vi "tester CE14(APIs).vi"() -> ()   [LabVIEW 2018, in "CE14_eMIC.lvlib"]
uses:
  CE14_eMIC.lvlib
  <vilib>/ErrorRing/Error Ring.xnode
panel:
  out "log":string
  out "output 1":dbl
  out "kvar (x.xxxx*kvar)":string
  out "kW (x.xxxx*kW)":string
  out "PF(x.xxx)":string
  out "freq (xx.xxHz)":string
  out "voltage(xxx.xx*V)":string
  out "Current (x.xx Amps)":string
  in  "VISA resource name":refnum<visa-resource-name>="COM12"
  out "success":bool
  in  "kvar":bool
  in  "kW":bool
  in  "pf":bool
  in  "Freq":bool
  in  "voltage":bool
  in  "curr":bool
  in  "stop":bool
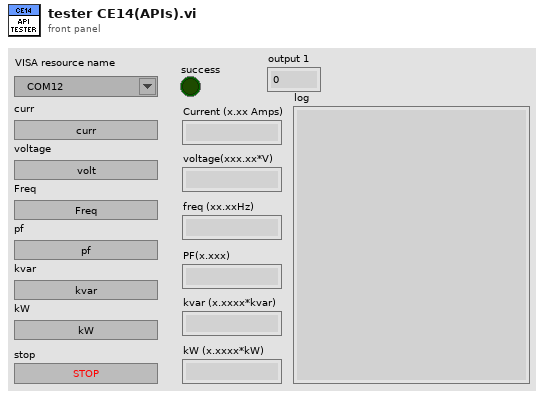
[diagram p1: front panel]
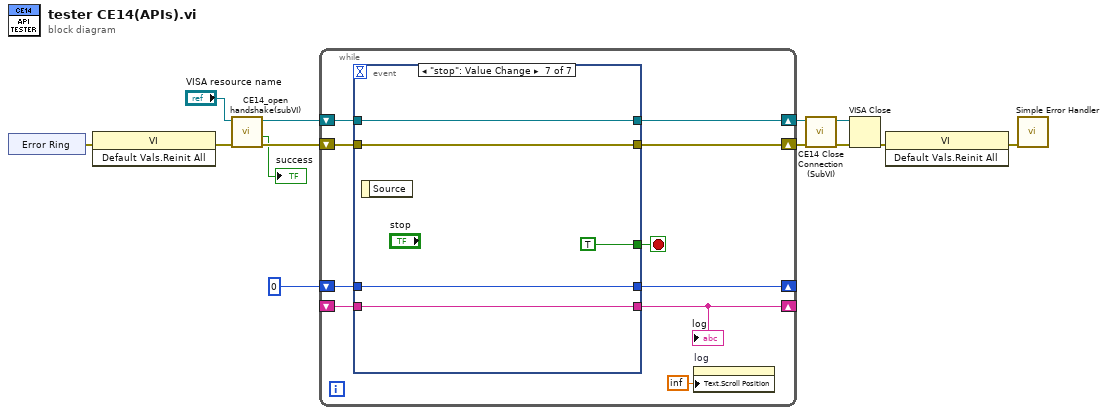
[diagram p0: block diagram]
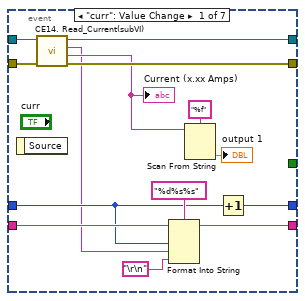
[diagram p2: hidden frame]
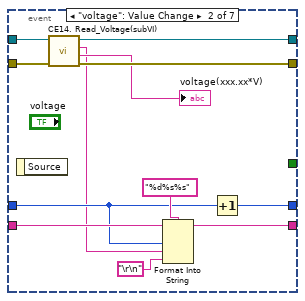
[diagram p3: hidden frame]
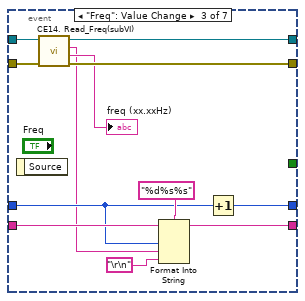
[diagram p4: hidden frame]
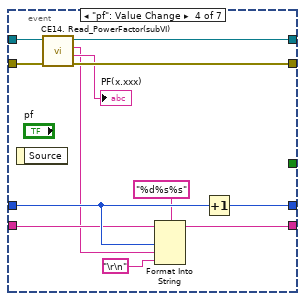
[diagram p5: hidden frame]
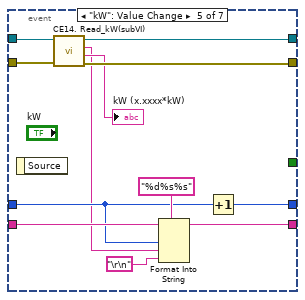
[diagram p6: hidden frame]
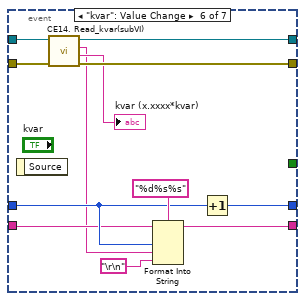
[diagram p7: hidden frame]
diagram:
  n1 = xnode "Error Ring"() -> ("error out"=w13:errorcluster)
  n2 = invoke class="VI" method="Default Vals.Reinit All"(error in=w13) -> (error out=w11:errorcluster)  [unwired: 2 in, 2 out]
  n3 = call "CE14_open handshake(subVI).vi"("error in(no error)"=w11, "VISA resource name"="VISA resource name") -> ("error out"=w10:errorcluster, "success"=→"success":bool, "VISA resource name 2"=w9:refnum<visa-resource-name>)  [unwired: 6 in, 1 out]
  n4 = while {
    shift-right: [w22] -> w6
    shift-left: w10 -> [w23]
    shift-right: [w19] -> w2
    shift-left: w9 -> [w20]
    shift-right: [w18] -> _
    shift-left: _ -> [w17]
    shift-right: [w15] -> _
    shift-left: 0 -> [w16]
    stop <- w21 stop-if-true
    n5 = event shown="[6] \"stop\": Value Change" {
      selector: _ -> [_ _ _ _ _ _ _]
      dyn-events: _ -> [_ _ _ _ _ _ _]
      timeout: _ -> [_ _ _ _ _ _ _]
      tunnel: w20 -> [w37 w49 w61 w72 w84 w97 w101]
      tunnel: w23 -> [w36 w48 w60 w73 w85 w96 w102]
      tunnel: [w34 w47 w59 w71 w83 w95 w102] -> w22
      tunnel: [_ _ _ _ _ _ TRUE] -> w21
      tunnel: [w35 w46 w58 w70 w82 w94 w101] -> w19
      tunnel: [w31 w38 w51 w65 w77 w88 w99] -> w18
      tunnel: w17 -> [w30 w42 w54 w66 w76 w89 w99]
      tunnel: w16 -> [w27 w41 w52 w67 w75 w90 w98]
      tunnel: [w26 w43 w53 w64 w78 w87 w98] -> w15
      event "curr": Value Change {
        n6 = event-data() -> ()  [unwired: 1 in, 1 out]
        n7 = call "CE14. Read_Current(subVI).vi"("error in (no error)"=w36, "VISA resource name"=w37) -> ("error out"=w34:errorcluster, "Current (x.xx Amps)"=w28:string, "received msg"=w25:string, "VISA resource name out"=w35:refnum<visa-resource-name>)  [unwired: 6 in]
        "Current (x.xx Amps)" <- w28
        n8 = Format Into String(format string="%d%s%s", initial string=w30, w27, w25, "\r\n") -> (resulting string=w31:string)  [unwired: 1 in, 1 out]
        n9 = Scan From String(format string="%f", input string=w28) -> (output 1=→"output 1":dbl)  [unwired: 3 in, 3 out]
        n10 = Increment(x=w27) -> (x+1=w26:i32)
      }
      event "voltage": Value Change {
        n11 = event-data() -> ()  [unwired: 1 in, 1 out]
        n12 = call "CE14. Read_Voltage(subVI).vi"("error in (no error)"=w48, "VISA resource name"=w49) -> ("error out"=w47:errorcluster, "voltage(xxx.xx*V)"=→"voltage(xxx.xx*V)":string, "read buffer"=w40:string, "VISA resource name out"=w46:refnum<visa-resource-name>)  [unwired: 6 in]
        n13 = Format Into String(format string="%d%s%s", initial string=w42, w41, w40, "\r\n") -> (resulting string=w38:string)  [unwired: 1 in, 1 out]
        n14 = Increment(x=w41) -> (x+1=w43:i32)
      }
      event "Freq": Value Change {
        n15 = event-data() -> ()  [unwired: 1 in, 1 out]
        n16 = call "CE14. Read_Freq(subVI).vi"("error in (no error)"=w60, "VISA resource name"=w61) -> ("error out"=w59:errorcluster, "freq (xx.xxHz)"=→"freq (xx.xxHz)":string, "read buffer"=w50:string, "VISA resource name out"=w58:refnum<visa-resource-name>)  [unwired: 6 in]
        n17 = Format Into String(format string="%d%s%s", initial string=w54, w52, w50, "\r\n") -> (resulting string=w51:string)  [unwired: 1 in, 1 out]
        n18 = Increment(x=w52) -> (x+1=w53:i32)
      }
      event "pf": Value Change {
        n19 = event-data() -> ()  [unwired: 1 in, 1 out]
        n20 = call "CE14. Read_PowerFactor(subVI).vi"("error in (no error)"=w73, "VISA resource name"=w72) -> ("error out"=w71:errorcluster, "PF(x.xxx)"=→"PF(x.xxx)":string, "read buffer"=w62:string, "VISA resource name out"=w70:refnum<visa-resource-name>)  [unwired: 6 in]
        n21 = Format Into String(format string="%d%s%s", initial string=w66, w67, w62, "\r\n") -> (resulting string=w65:string)  [unwired: 1 in, 1 out]
        n22 = Increment(x=w67) -> (x+1=w64:i32)
      }
      event "kW": Value Change {
        n23 = event-data() -> ()  [unwired: 1 in, 1 out]
        n24 = call "CE14. Read_kW(subVI).vi"("error in (no error)"=w85, "VISA resource name"=w84) -> ("error out"=w83:errorcluster, "kW (x.xxxx*kW)"=→"kW (x.xxxx*kW)":string, "read buffer"=w74:string, "VISA resource name out"=w82:refnum<visa-resource-name>)  [unwired: 6 in]
        n25 = Format Into String(format string="%d%s%s", initial string=w76, w75, w74, "\r\n") -> (resulting string=w77:string)  [unwired: 1 in, 1 out]
        n26 = Increment(x=w75) -> (x+1=w78:i32)
      }
      event "kvar": Value Change {
        n27 = event-data() -> ()  [unwired: 1 in, 1 out]
        n28 = call "CE14. Read_kvar(subVI).vi"("error in (no error)"=w96, "VISA resource name"=w97) -> ("error out"=w95:errorcluster, "kvar (x.xxxx*kvar)"=→"kvar (x.xxxx*kvar)":string, "read buffer"=w86:string, "VISA resource name out"=w94:refnum<visa-resource-name>)  [unwired: 6 in]
        n29 = Format Into String(format string="%d%s%s", initial string=w89, w90, w86, "\r\n") -> (resulting string=w88:string)  [unwired: 1 in, 1 out]
        n30 = Increment(x=w90) -> (x+1=w87:i32)
      }
      event "stop": Value Change {
        n31 = event-data() -> ()  [unwired: 1 in, 1 out]
      }
    }
    "log" <- w18
    n32 = property on="log" class="Str"("Text.Scroll Position"=inf) -> ()  [unwired: 2 in, 2 out]
  }
  n33 = call "CE14 Close Connection (SubVI).vi"("error in (no error)"=w6, "VISA Refnum in"=w2) -> ("error out"=w5:errorcluster, "VISA Refnum out"=w4:refnum<visa-resource-name>)  [unwired: 8 in]
  n34 = VISA Close(VISA resource name=w4, error in (no error)=w5) -> (error out=w3:errorcluster)
  n35 = invoke class="VI" method="Default Vals.Reinit All"(error in=w3) -> (error out=w12:errorcluster)  [unwired: 2 in, 2 out]
  n36 = call <vilib>:"Simple Error Handler.vi"("error in (no error)"=w12) -> ()  [unwired: 4 in, 5 out]
